vi "DtOLReadMultipleSingleU16.vi"(5 "Number Chan to Read":u32, 7 "OnlyReadAvailable":bool, 8 "error in (no error)":errorcluster, 9 "Timeout":dbl=10.0, 11 "Task in":i32) -> (0 "error out":errorcluster, 1 "Num Samples Per Channel Read":u32, 2 "2D Data out":u16[][](array[numeric]), 3 "Task out":i32, 4 "Num Channels Read":u32)   [LabVIEW 2022 SP3]
doc: "Reads a single sample from multiple virtual channels of a task you specify, and returns the data as a two-dimensional array of unsigned 16-bit numbers. This VI is typically used with analog input tasks that use the DtOLTiming (Input - Set Timing) VI."
uses:
  DtLvLink.lvlib
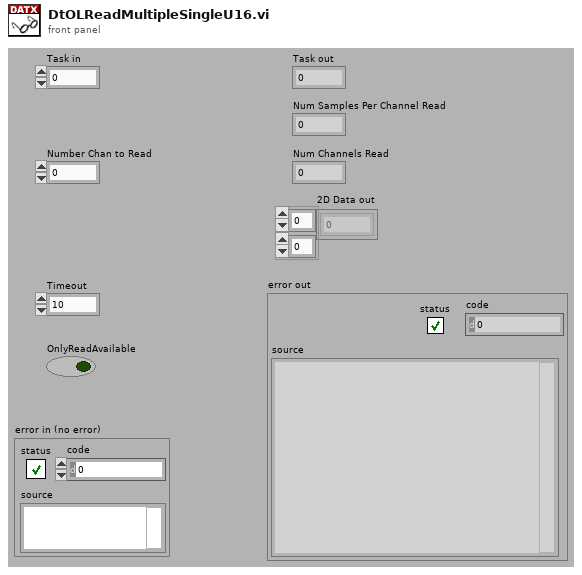
[diagram p1: front panel]
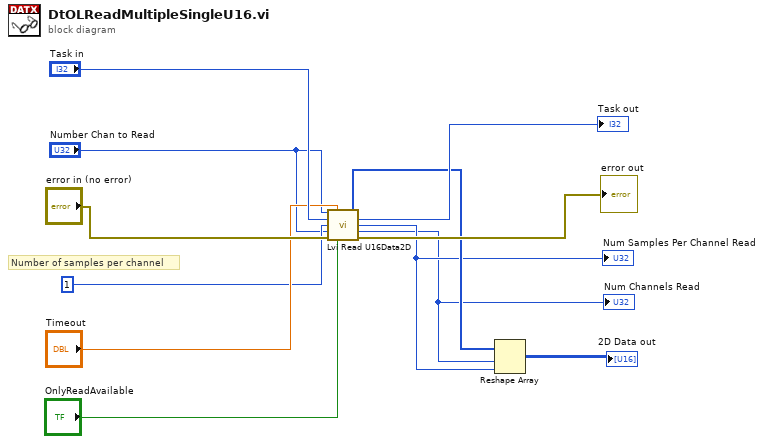
[diagram p0: block diagram]
diagram:
  # "Number of samples per channel"
  n1 = call "Lvi Read U16Data2D.vi"("DataBufSize"="Number Chan to Read", "timeout"="Timeout", "TaskRef"="Task in", "PointsPerChan"=1, "NumChansToRead"="Number Chan to Read", "error in (no error)"="error in (no error)", "OnlyReadAvailable"="OnlyReadAvailable") -> ("DataBuf"=w6:u16[], "TaskRef out"=→"Task out":i32, "PointsPerChan out"=w4:u32, "NumChansToRead out"=w3:u32, "error out"=→"error out":errorcluster)  [unwired: 2 in, 2 out]
  "Num Samples Per Channel Read" <- w4
  "Num Channels Read" <- w3
  n2 = Reshape Array "Reshape Array"(w6, w3, w4) -> (→"2D Data out":u16[][])
